vi "aggregator - Arrays.vi"(6 "first time":bool=TRUE, 7 "requested size":i32=1, 10 "Array in":cdb[](array[numeric])) -> (3 "Array":cdb[](array[numeric]))   [LabVIEW 2010]
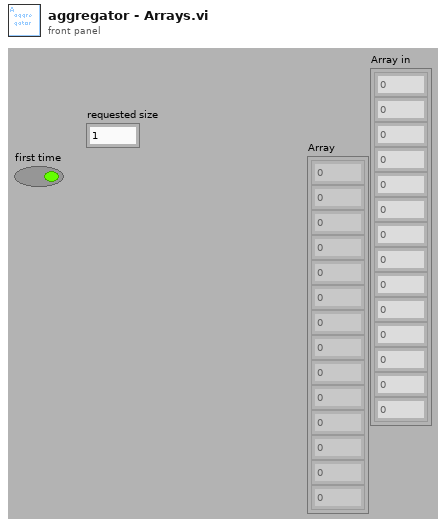
[diagram p1: front panel]
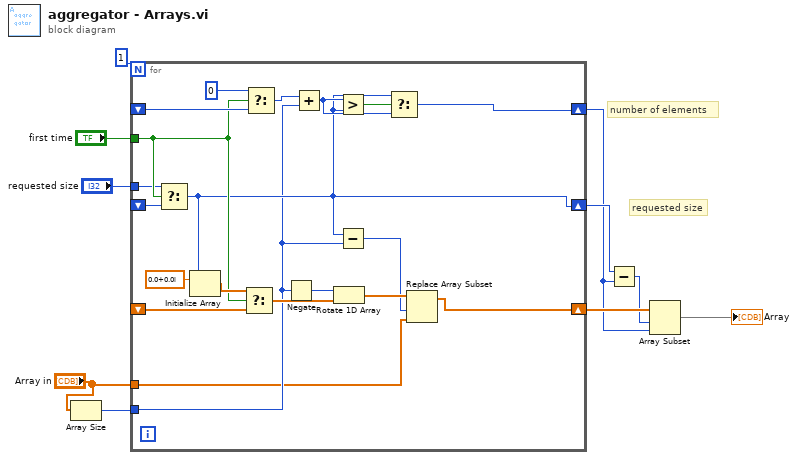
[diagram p0: block diagram]
diagram:
  # "requested size"
  # "number of elements"
  n1 = Array Size(array="Array in") -> (size(s)=w2:i32)
  n2 = for {
    N: 1 -> [_]
    tunnel: "first time" -> [w22]
    shift-right: [w27] -> w3
    shift-left: _ -> [w29]
    tunnel: "requested size" -> [w21]
    shift-right: [w13] -> w7
    shift-left: _ -> [w26]
    shift-right: [w16] -> w5
    shift-left: _ -> [w20]
    tunnel: w2 -> [w15]
    tunnel: "Array in" -> [w11]
    n3 = Select(t=w21, s=w22, f=w20) -> (s? t:f=w16:i32)
    n4 = Initialize Array(cdb 0.0+0.0i, w16) -> (w23:cdb[])
    n5 = Select(t=w23, s=w22, f=w26) -> (s? t:f=w25:cdb[])
    n6 = Select(t=0, s=w22, f=w29) -> (s? t:f=w19:i32)
    n7 = Negate(x=w15) -> (-x=w17:i32)
    n8 = Add(x=w19, y=w15) -> (x+y=w18:i32)
    n9 = Rotate 1D Array(1:w25, 2:w17) -> (0:w14:cdb[])
    n10 = Greater?(x=w18, y=w16) -> (0:w28:bool)
    n11 = Subtract(x=w16, y=w15) -> (x-y=w12:i32)
    n12 = Select(t=w16, s=w28, f=w18) -> (s? t:f=w27:i32)
    n13 = Replace Array Subset(array=w14, new element=w11, index=w12) -> (w13:cdb[])
  }
  n14 = Subtract(x=w5, y=w3) -> (x-y=w4:i32)
  n15 = Array Subset(array=w7, index=w4, length=w3) -> (→"Array":cdb[])
